vi "Write Lockin parameters.vi"(8 "error in (no error)":errorcluster, 10 "Lockin parameters":T1={"Frequency"=0.0, "Phase"=0.0, "Syncronous"=FALSE, "Points per sine wave"=0, "DDS"=FALSE, "Frequency word"=0, "Phase word"=0, "DDS modulus"=15120, "DDS clock"=125000000.0} {"DDS clock" format="%_17pHz"; "DDS modulus" format="0x%x (%d)"; "Phase" format="%#_gdeg"; "Frequency" format="%_17pHz"}, 11 "Lock-in Detector in":refnum<class "Lock-in Detector.lvclass">) -> (0 "error out":errorcluster, 3 "Lock-in Detector out":refnum<class "Lock-in Detector.lvclass">)   [LabVIEW 2020, in "Lock-in Detector.lvclass"]
uses:
  Lock-in Detector.lvclass
  Lockin Parameters.ctl
  Lock-in Detector.lvclass/Lock-in Detector.ctl
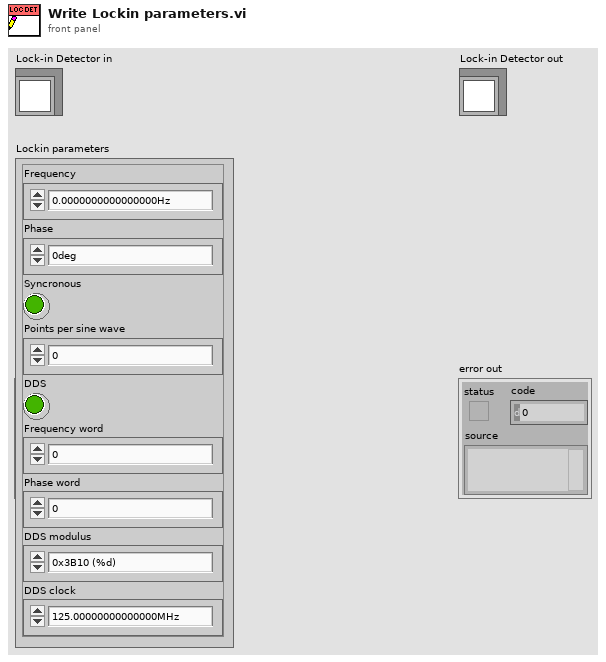
[diagram p1: front panel]
types:
  T1 = typedef "Lockin Parameters.ctl" = cluster{"Frequency":dbl, "Phase":dbl, "Syncronous":bool, "Points per sine wave":i32, "DDS":bool, "Frequency word":u32, "Phase word":u32, "DDS modulus":i64, "DDS clock":dbl}
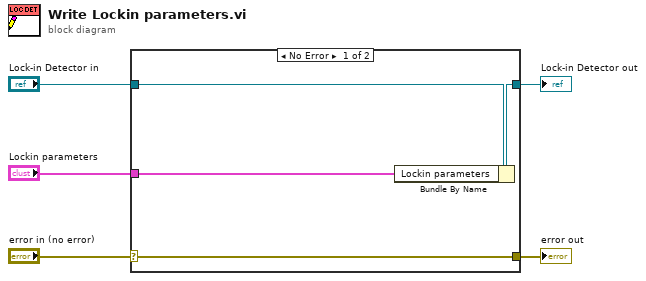
[diagram p0: block diagram]
diagram:
  n1 = case shown="No Error" "error in (no error)" {
    selector: "error in (no error)" -> [w9 w10]
    tunnel: [w9 w10] -> w4
    tunnel: [w7 w11] -> w2
    tunnel: "Lock-in Detector in" -> [w8 w11]
    tunnel: "Lockin parameters" -> [w6 _]
    frame No Error {
      n2 = Bundle By Name(cluster=w8, "Lockin parameters"=w6) -> (w7:refnum<class "Lock-in Detector.lvclass">)
    }
    frame Error {
    }
  }
  "error out" <- w4
  "Lock-in Detector out" <- w2
